vi "ma_resample single-shot (linear interpolation).vi"(6 "#elements":i32, 8 "error in":errorcluster, 9 "t0":timestamp format="%<%.4X>T", 10 "dt":dbl=1.0 format="%.2p", 11 "waveform in":waveform(dbl)) -> (0 "error out":errorcluster, 3 "resampled waveform out":waveform(dbl))   [LabVIEW 2020, in "NI_MAPro.lvlib"]
doc: "This VI re-samples an unevenly sampled input signal to an evenly sampled waveform according to specified t0 and dt. If the specified t0 value is less than the first value of input X-array (that is the timestamp of the first input sample), then the VI will coerce t0 to the first valid value (greater than X(0)) that also fulfill the relation:\n\nT0_adjusted - t0_in = n * dt_in\n\nThis guarranty that any later comparison of waveforms will be correct with repsect to absolute time."
uses:
  NI_MAPro.lvlib
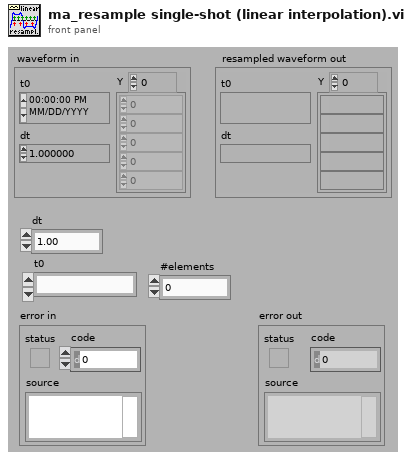
[diagram p1: front panel]
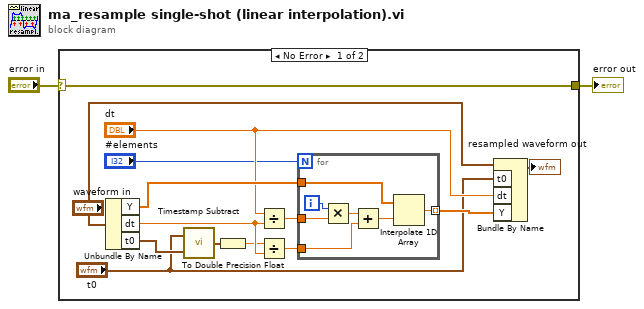
[diagram p0: block diagram]
diagram:
  n1 = case shown="No Error" "error in" {
    selector: "error in" -> [w7 w24]
    tunnel: [w7 w24] -> w1
    frame No Error {
      n2 = Unbundle By Name("waveform in") -> ("Y"=w14:dbl[], "dt"=w9:dbl, "t0"=w6:timestamp)
      n3 = call "Timestamp Subtract.vi"("y"=w6, "x"="t0") -> ("x - y"=w3:timestamp)
      n4 = To Double Precision Float(number=w3) -> (double precision float=w4:dbl)
      n5 = Divide(x="dt", y=w9) -> (x/y=w12:dbl)
      n6 = Divide(x=w4, y=w9) -> (x/y=w11:dbl)
      n7 = for {
        N: "#elements" -> [_]
        tunnel: w12 -> [w22]
        tunnel: w14 -> [w18]
        tunnel: [w17] -> w13 mode=indexing
        tunnel: w11 -> [w20]
        i -> [w23]
        n8 = Multiply(x=w23, y=w22) -> (x*y=w21:dbl)
        n9 = Add(x=w21, y=w20) -> (x+y=w19:dbl)
        n10 = Interpolate 1D Array(1:w19, 2:w18) -> (0:w17:dbl)
      }
      n11 = Bundle By Name(cluster="waveform in", "t0"="t0", "dt"="dt", "Y"=w13) -> (→"resampled waveform out":waveform(dbl))
    }
    frame Error {
    }
  }
  "error out" <- w1
